vi "DataFrom_ini (SubVI).vi"(8 "error in (no error)":errorcluster, 10 "UUT":string, 11 "appended path":path) -> (0 "error out":errorcluster, 1 "FileName":string, 2 "Next SN":i32, 3 "UUT SoftwareVer":string, 5 "PN":string)   [LabVIEW 2017]
uses:
  <vilib>/Utility/config.llb/Read Key (String).vi
  <vilib>/Utility/config.llb/NI_LVConfig.lvlib
panel:
  out "found?":bool
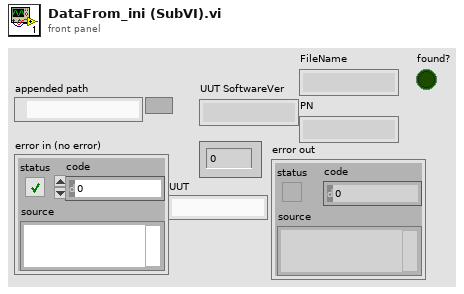
[diagram p1: front panel]
types:
  T1 = typedef "NI_LVConfig.lvlib/Config Data RefNum.ctl" = refnum<k1>
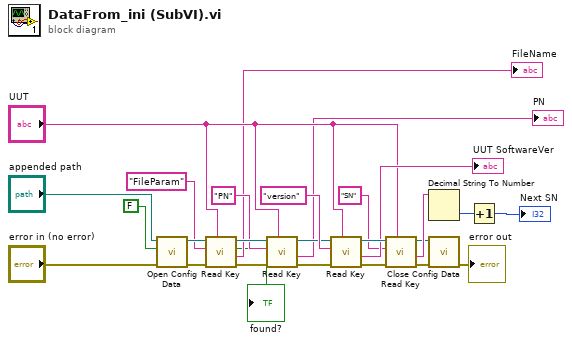
[diagram p0: block diagram]
diagram:
  n1 = call <vilib>:"Open Config Data.vi"("error in (no error)"="error in (no error)", "create file if necessary (T)"=FALSE, "configuration file path"="appended path") -> ("error out"=w8:errorcluster, "refnum"=w13:T1)  [unwired: 7 out]
  n2 = call-poly <vilib>:"Read Key.vi"("section"="UUT", "error in (no error)"=w8, "key"="FileParam", "refnum"=w13) -> ("error out"=w9:errorcluster, "value"=→"FileName":string, "found?"=→"found?":bool, "refnum out"=w12:T1)  [unwired: 2 in, 2 out]
  n3 = call-poly <vilib>:"Read Key.vi"("section"="UUT", "error in (no error)"=w9, "key"="PN", "refnum"=w12) -> ("error out"=w10:errorcluster, "value"=→"PN":string, "refnum out"=w11:T1)  [unwired: 2 in, 3 out]
  n4 = call-poly <vilib>:"Read Key.vi"("section"="UUT", "error in (no error)"=w10, "key"="version", "refnum"=w11) -> ("error out"=w17:errorcluster, "value"=→"UUT SoftwareVer":string, "refnum out"=w18:T1)  [unwired: 2 in, 3 out]
  n5 = call-poly <vilib>:"Read Key.vi"("section"="UUT", "error in (no error)"=w17, "key"="SN", "refnum"=w18) -> ("error out"=w22:errorcluster, "value"=w24:string, "refnum out"=w23:T1)  [unwired: 2 in, 3 out]
  n6 = Decimal String To Number(string=w24) -> (number=w26:i32)  [unwired: 2 in, 1 out]
  n7 = call <vilib>:"Close Config Data.vi"("error in (no error)"=w22, "refnum"=w23) -> ("error out"=→"error out":errorcluster)  [unwired: 8 in, 1 out]
  n8 = Increment(x=w26) -> (x+1=→"Next SN":i32)
